vi "predict_proba.vi"(8 "error in (no error)":errorcluster, 11 "VotingClassifier in":refnum<class "VotingClassifier.lvclass">) -> (0 "error out":errorcluster, 2 "T":dbl[][](array[numeric]), 3 "VotingClassifier out":refnum<class "VotingClassifier.lvclass">)   [LabVIEW 2020, in "VotingClassifier.lvclass"]
uses:
  VotingClassifier.lvclass
  C:/Users/cipop/TDF Dropbox/2_Technologies de France/1 - Services et Etudes/PLAIY/2 - DEV/PLAIYLAB/code/Python/Python.lvclass
  C:/Users/cipop/TDF Dropbox/2_Technologies de France/1 - Services et Etudes/PLAIY/2 - DEV/PLAIYLAB/code/Model/Model.lvclass
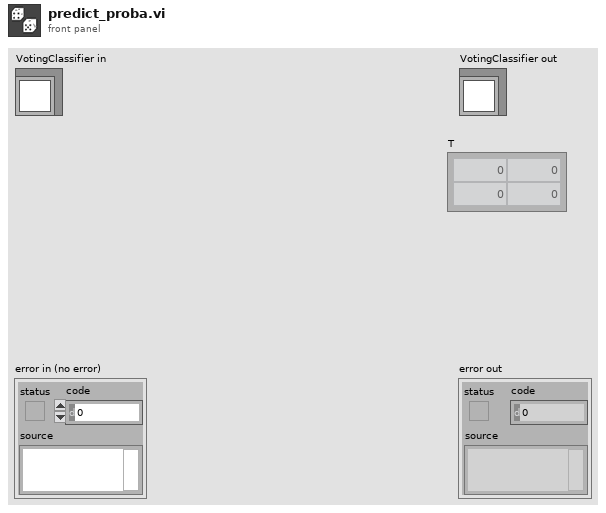
[diagram p1: front panel]
types:
  T1 = typedef "data.ctl" = cluster{"name":string, "X":dbl[][]}
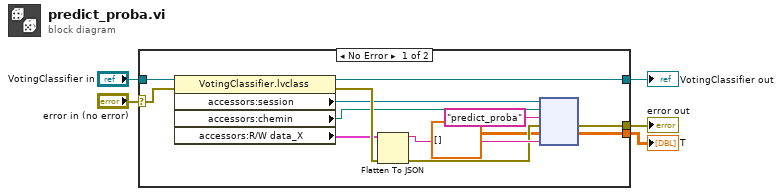
[diagram p0: block diagram]
diagram:
  n1 = case shown="No Error" "error in (no error)" {
    selector: "error in (no error)" -> [w16 w20]
    tunnel: [w17 w20] -> w3
    tunnel: [w9 w19] -> w4
    tunnel: "VotingClassifier in" -> [w8 w19]
    tunnel: [w6 _] -> w2
    frame No Error {
      n2 = property class="VotingClassifier.lvclass"(reference=w8, error in=w16) -> (reference out=w9:refnum<class "VotingClassifier.lvclass">, error out=w14:errorcluster, "accessors:session"=w11:refnum<k35>, "accessors:chemin"=w10:path, "accessors:R/W data_X"=w12:T1)
      n3 = Flatten To JSON(anything=w12, error in (no error)=w14) -> (JSON string=w15:string, 11:w13:errorcluster)  [unwired: 1 in]
      n4 = node(w11, w10, "predict_proba" ("nom de la fonction"), w13, dbl[][] [], w15) -> (w17:errorcluster, w6:dbl[][])  [unwired: 1 in, 3 out]
    }
    frame Error {
    }
  }
  "error out" <- w3
  "VotingClassifier out" <- w4
  "T" <- w2
